vi "Run Contest.vi"() -> ()   [LabVIEW 2014]
uses:
  Participant.ctl
  Problem.ctl
  State Machine.ctl
  User Score Update.ctl
  Change Detect/Change Detect Int.vi
  Change Detect/Change Detect Boolean.vi
panel:
  in  "Update Ratings":bool
  in  "Early Finish":bool
  in  "Export Results":bool
  in  "Participant Names":string[](array[string])
  in  "Contest Length (hours)":dbl
  in  "Problem E Base Value":dbl=2500.0
  in  "Problem D Base Value":dbl=2000.0
  in  "Problem C Base Value":dbl=1500.0
  in  "Problem B Base Value":dbl=1000.0
  in  "Problem A Base Value":dbl=500.0
  in  "OK Button":bool
  in  "Problem":T1
  in  "Participant":string
  in  "At Time Remaining":dbl=3600.0
  out "Participant Status":T2[](array[typedef])
  in  "Participants":dbl
  in  "Contest Start":bool
  out "Time Remaining":u32
  out "Contest Indicator":bool
  out "Problem E Current Value":dbl
  out "Problem D Current Value":dbl
  out "Problem C Current Value":dbl
  out "Problem B Current Value":dbl
  out "Problem A Current Value":dbl
  # "You must export before starting a new Contest"
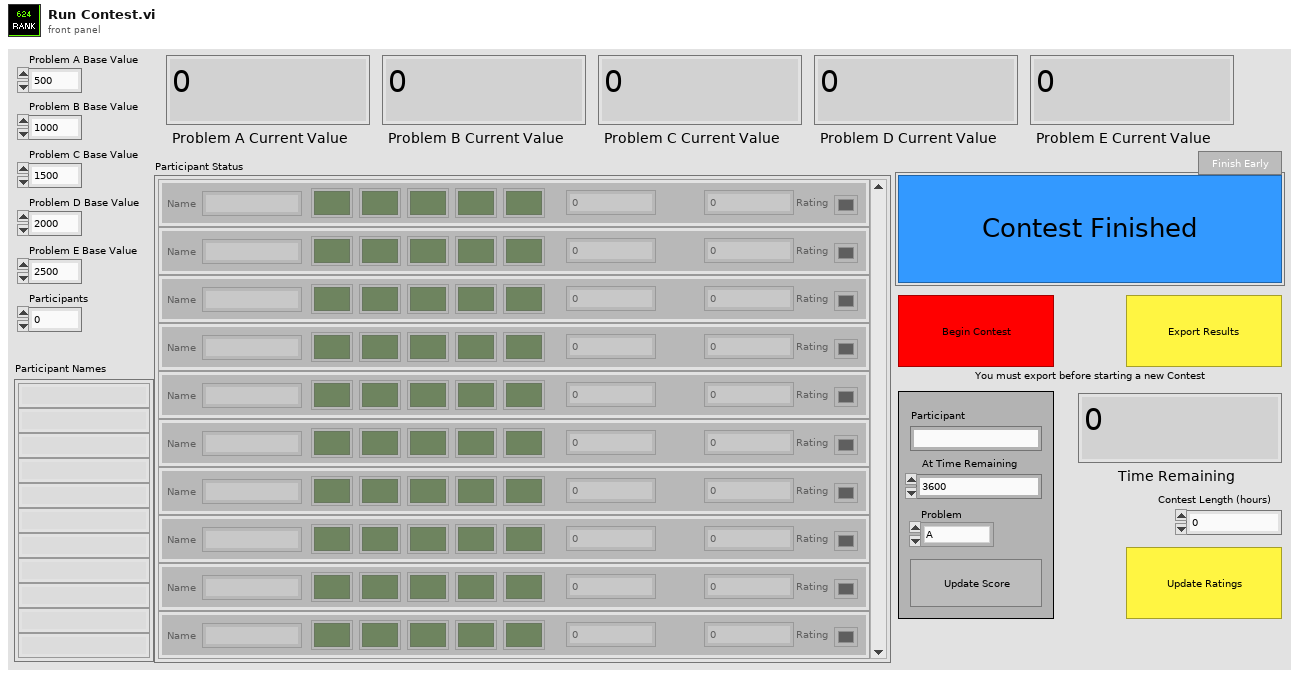
[diagram p1: front panel]
types:
  T1 = typedef "Problem.ctl" = enum16{"A", "B", "C", "D", "E"}
  T2 = typedef "Participant.ctl" = cluster{"Name":string, "A":bool, "Score":dbl, "B":bool, "C":bool, "D":bool, "E":bool, "Rating":dbl, "Color Box":u32}
  T3 = typedef "State Machine.ctl" = enum16{"Finish Contest", "Run Contest", "Begin Contest", "Wait for Start"}
  T4 = typedef "User Score Update.ctl" = cluster{"Score":dbl, "Name":string}
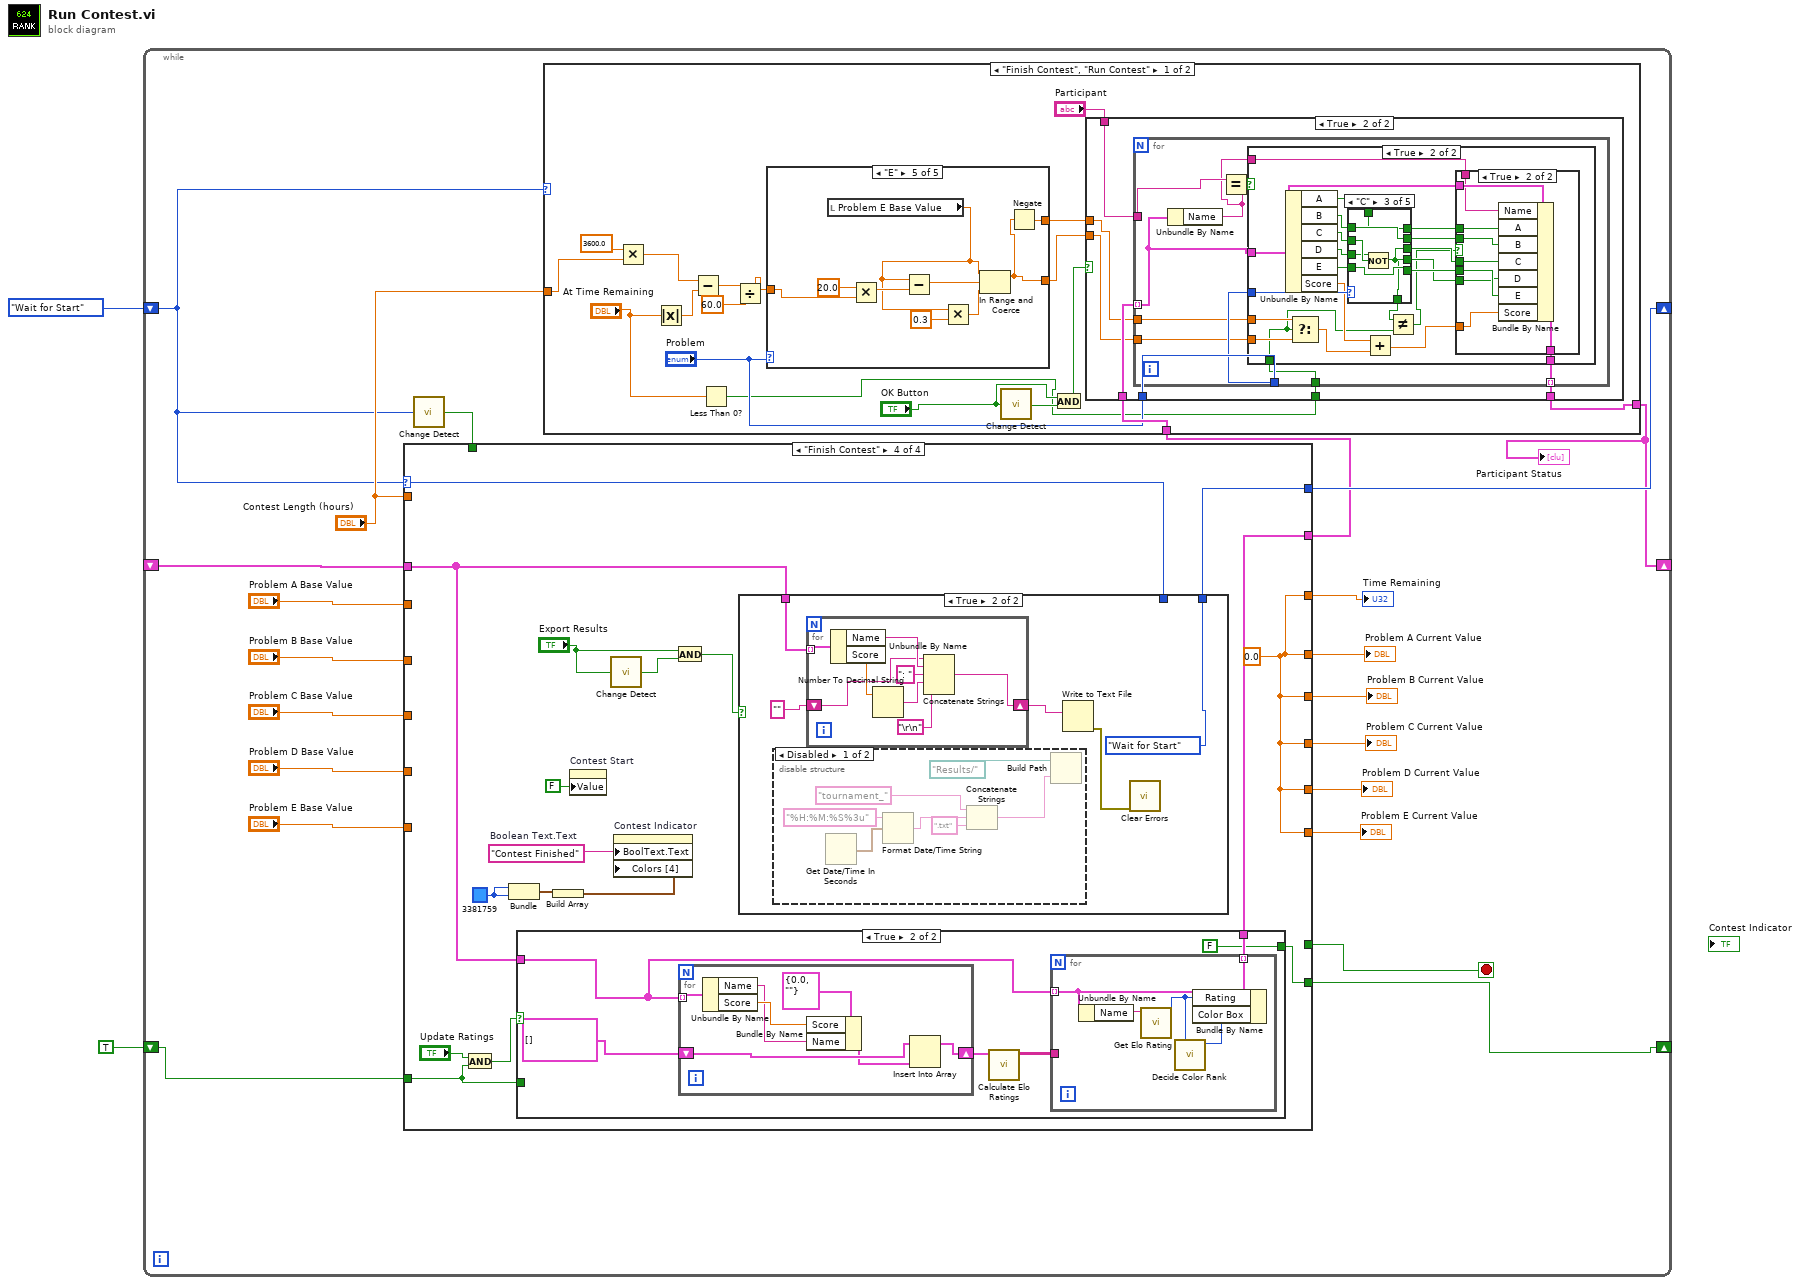
[diagram p0: block diagram]
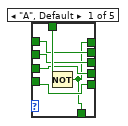
[diagram p5: hidden frame]
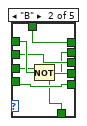
[diagram p6: hidden frame]
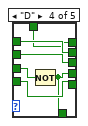
[diagram p7: hidden frame]
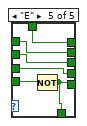
[diagram p8: hidden frame]
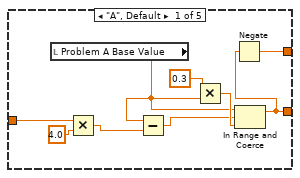
[diagram p9: hidden frame]
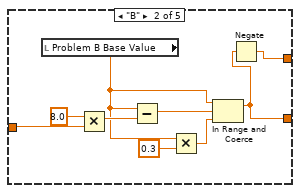
[diagram p10: hidden frame]
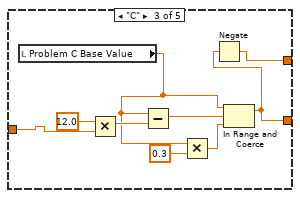
[diagram p11: hidden frame]
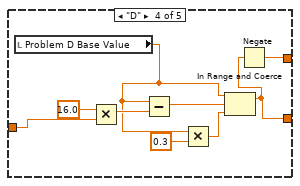
[diagram p12: hidden frame]
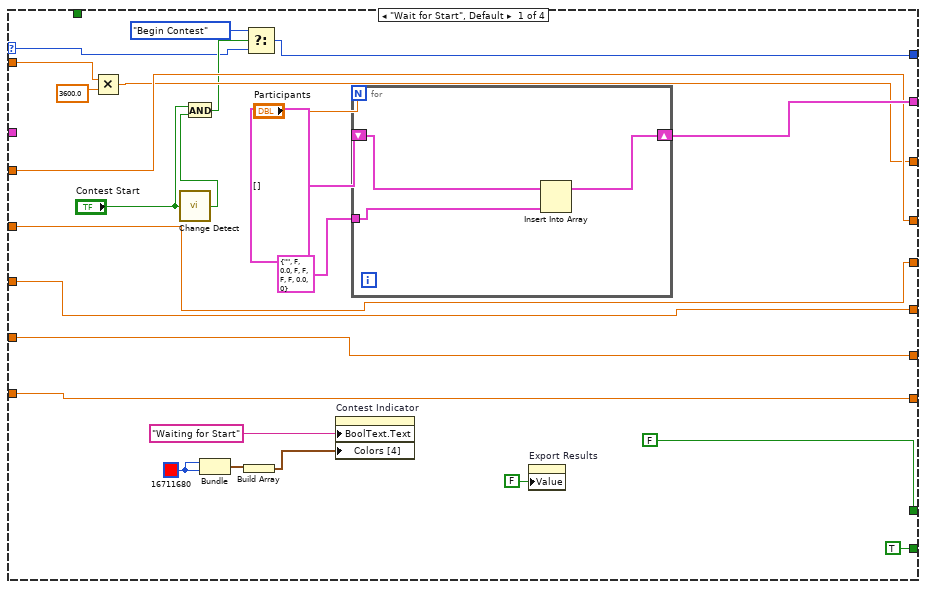
[diagram p14: hidden frame]
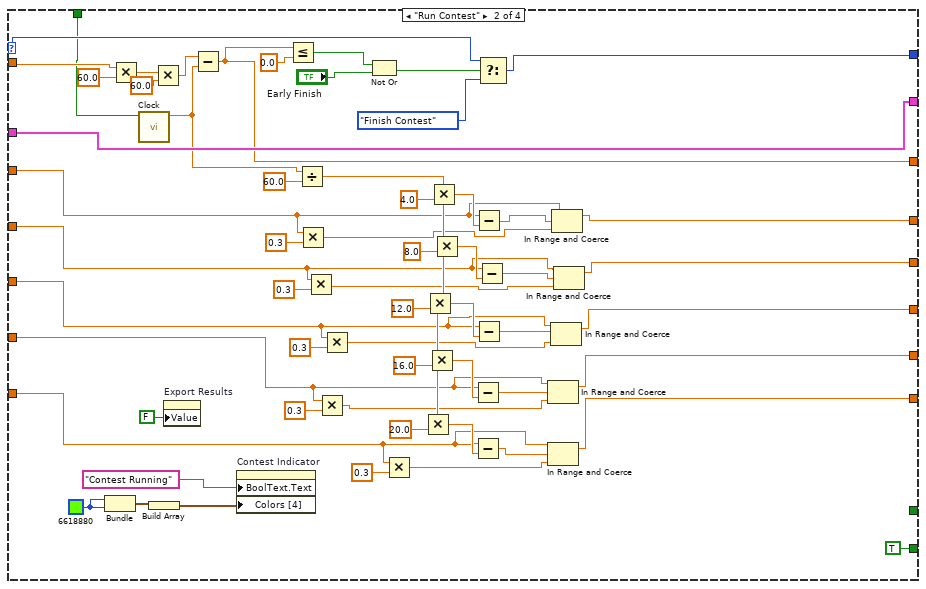
[diagram p15: hidden frame]
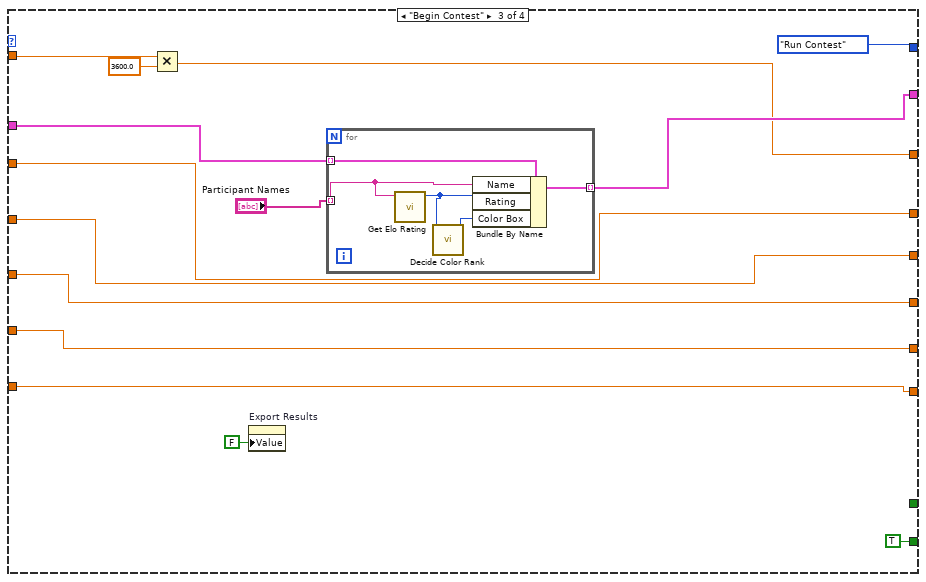
[diagram p16: hidden frame]
diagram:
  n1 = while {
    shift-right: [w6] -> _
    shift-left: _ -> [w22]
    shift-right: [w16] -> _
    shift-left: State_Machine."Wait for Start" -> [w5]
    shift-right: [w3] -> _
    shift-left: TRUE -> [w4]
    stop <- w23 stop-if-true
    n2 = call-poly "Change Detect.vi"("In"=w5) -> ("Changed?"=w9:bool)
    n3 = case shown="\"Finish Contest\"" w5 {
      selector: w5 -> [w170 w244 _ w282]
      tunnel: [FALSE _ _ _] -> w23
      tunnel: [w188 w242 w266 w278] -> w7
      tunnel: w22 -> [_ w242 w267 w279]
      tunnel: "Problem A Base Value" -> [w179 w227 w264 _]
      tunnel: "Problem B Base Value" -> [w180 w219 w263 _]
      tunnel: "Problem C Base Value" -> [w181 w216 w262 _]
      tunnel: "Problem D Base Value" -> [w182 w211 w261 _]
      tunnel: "Problem E Base Value" -> [w183 w208 w260 _]
      tunnel: "Contest Length (hours)" -> [w178 w246 w259 _]
      tunnel: [w169 w243 State_Machine."Run Contest" w281] -> w16
      tunnel: [w179 w228 w264 w286] -> w15
      tunnel: [w180 w217 w263 w286] -> w14
      tunnel: [w181 w213 w262 w286] -> w13
      tunnel: [w182 w209 w261 w286] -> w12
      tunnel: [w183 w205 w260 w286] -> w11
      tunnel: [w176 w204 w257 w286] -> w10
      tunnel: w9 -> [_ w203 _ _]
      tunnel: w4 -> [_ _ _ w274]
      tunnel: [TRUE TRUE TRUE w275] -> w3
      frame "Wait for Start", Default {
        w186 = u32 16711680
        n4 = Multiply(x=w178, y=3600.0) -> (x*y=w176:dbl)
        n5 = call-poly "Change Detect.vi"("In"="Contest Start") -> ("Changed?"=w173:bool)
        n6 = And(x="Contest Start", y=w173) -> (x .and. y?=w172:bool)
        n7 = Bundle(w186, w186) -> (w185:cluster{u32, u32})  [unwired: 1 in]
        n8 = Build Array(w185) -> (w184:cluster{u32, u32}[])
        n9 = Select(t=State_Machine."Begin Contest", s=w172, f=w170) -> (s? t:f=w169:T3)
        n10 = property on="Contest Indicator" class="Bool (strict)"("BoolText.Text"="Waiting for Start" ("Boolean Text.Text"), "Colors [4]"=w184) -> ()  [unwired: 2 in, 2 out]
        n11 = for {
          N: "Participants" -> [_]
          shift-right: [w195] -> w188
          shift-left: T2[] [] ("array") -> [w194]
          tunnel: T2 {"Name"="", "A"=FALSE, "Score"=0.0, "B"=FALSE, "C"=FALSE, "D"=FALSE, "E"=FALSE, "Rating"=0.0, "Color Box"=0} ("Participant") -> [w193]
          n12 = Insert Into Array(array=w194, new element=w193) -> (w195:T2[])  [unwired: 1 in]
        }
        n13 = property on="Export Results" class="Bool (strict)"("Value"=FALSE ("Export Results")) -> ()  [unwired: 2 in, 2 out]
      }
      frame "Run Contest" {
        w253 = u32 6618880
        n14 = Bundle(w253, w253) -> (w252:cluster{u32, u32})  [unwired: 1 in]
        n15 = Multiply(x=w246, y=60.0) -> (x*y=w248:dbl)
        n16 = call "Clock.vi"("Reset?"=w203) -> ("Time Elapsed"=w202:dbl)  [unwired: 10 in]
        n17 = Build Array(w252) -> (w251:cluster{u32, u32}[])
        n18 = Multiply(x=w248, y=60.0) -> (x*y=w250:dbl)
        n19 = property on="Export Results" class="Bool (strict)"("Value"=FALSE ("Export Results")) -> ()  [unwired: 2 in, 2 out]
        n20 = Subtract(x=w250, y=w202) -> (x-y=w204:dbl)
        n21 = property on="Contest Indicator" class="Bool (strict)"("BoolText.Text"="Contest Running" ("Boolean Text.Text"), "Colors [4]"=w251) -> ()  [unwired: 2 in, 2 out]
        n22 = Less Or Equal?(x=w204, y=0.0) -> (x <= y?=w200:bool)
        n23 = Divide(x=w202, y=60.0) -> (x/y=w240:dbl)
        n24 = Multiply(x=w227, y=0.3) -> (x*y=w225:dbl)
        n25 = Multiply(x=w219, y=0.3) -> (x*y=w218:dbl)
        n26 = Multiply(x=w211, y=0.3) -> (x*y=w210:dbl)
        n27 = Multiply(x=w216, y=0.3) -> (x*y=w215:dbl)
        n28 = Not Or(1:"Early Finish", 2:w200) -> (0:w199:bool)
        n29 = Multiply(x=w208, y=0.3) -> (x*y=w207:dbl)
        n30 = Multiply(x=w240, y=20.0) -> (x*y=w230:dbl)
        n31 = Multiply(x=w240, y=12.0) -> (x*y=w232:dbl)
        n32 = Multiply(x=w240, y=16.0) -> (x*y=w231:dbl)
        n33 = Multiply(x=w240, y=4.0) -> (x*y=w234:dbl)
        n34 = Multiply(x=w240, y=8.0) -> (x*y=w233:dbl)
        n35 = Subtract(x=w211, y=w231) -> (x-y=w212:dbl)
        n36 = Subtract(x=w208, y=w230) -> (x-y=w206:dbl)
        n37 = Subtract(x=w227, y=w234) -> (x-y=w229:dbl)
        n38 = Subtract(x=w216, y=w232) -> (x-y=w214:dbl)
        n39 = Subtract(x=w219, y=w233) -> (x-y=w220:dbl)
        n40 = Select(t=w244, s=w199, f=State_Machine."Finish Contest") -> (s? t:f=w243:T3)
        n41 = In Range and Coerce(upper limit=w211, x=w212, lower limit=w210) -> (coerced(x)=w209:dbl)  [unwired: 1 out]
        n42 = In Range and Coerce(upper limit=w208, x=w206, lower limit=w207) -> (coerced(x)=w205:dbl)  [unwired: 1 out]
        n43 = In Range and Coerce(upper limit=w216, x=w214, lower limit=w215) -> (coerced(x)=w213:dbl)  [unwired: 1 out]
        n44 = In Range and Coerce(upper limit=w227, x=w229, lower limit=w225) -> (coerced(x)=w228:dbl)  [unwired: 1 out]
        n45 = In Range and Coerce(upper limit=w219, x=w220, lower limit=w218) -> (coerced(x)=w217:dbl)  [unwired: 1 out]
      }
      frame "Begin Contest" {
        n46 = Multiply(x=w259, y=3600.0) -> (x*y=w257:dbl)
        n47 = property on="Export Results" class="Bool (strict)"("Value"=FALSE ("Export Results")) -> ()  [unwired: 2 in, 2 out]
        n48 = for {
          tunnel: w267 -> [w273] mode=indexing
          tunnel: "Participant Names" -> [w271] mode=indexing
          tunnel: [w272] -> w266 mode=indexing
          n49 = call "Get Elo Rating.vi"("Name"=w271) -> ("Rating"=w270:i32)  [unwired: 10 in]
          n50 = call "Decide Color Rank.vi"("Numeric"=w270) -> ("Color Box"=w269:u32)  [unwired: 10 in]
          n51 = Bundle By Name(cluster=w273, "Name"=w271, "Rating"=w270, "Color Box"=w269) -> (w272:T2)
        }
      }
      frame "Finish Contest" {
        w286 = 0.0 ("Problem A Base Value")
        w289 = u32 3381759
        w287 = "Contest Finished"  # Boolean Text.Text
        n52 = And(x="Update Ratings", y=w274) -> (x .and. y?=w276:bool)
        n53 = Bundle(w289, w289) -> (w290:cluster{u32, u32})  [unwired: 1 in]
        n54 = case shown="True" w276 {
          tunnel: w279 -> [w292 w295]
          tunnel: [w292 w294] -> w278
          tunnel: [w291 FALSE] -> w275
          tunnel: w274 -> [w291 _]
          frame False {
          }
          frame True {
            n55 = for {
              tunnel: w295 -> [w310] mode=indexing
              shift-right: [w304] -> w297
              shift-left: T4[] [] ("Names") -> [w306]
              n56 = Unbundle By Name(w310) -> ("Name"=w307:string, "Score"=w308:dbl)
              n57 = Bundle By Name(cluster=T4 {"Score"=0.0, "Name"=""} ("Score Update"), "Score"=w308, "Name"=w307) -> (w305:T4)
              n58 = Insert Into Array(array=w306, new element=w305) -> (w304:T4[])  [unwired: 1 in]
            }
            n59 = call "Calculate Elo Ratings.vi"("Names"=w297) -> ("Rating 2D Array"=w296:string[][])  [unwired: 8 in, 2 out]
            n60 = for {
              tunnel: w296 -> [_]
              tunnel: w295 -> [w303] mode=indexing
              tunnel: [w301] -> w294 mode=indexing
              n61 = Unbundle By Name(w303) -> ("Name"=w302:string)
              n62 = call "Get Elo Rating.vi"("Name"=w302) -> ("Rating"=w300:i32)  [unwired: 10 in]
              n63 = call "Decide Color Rank.vi"("Numeric"=w300) -> ("Color Box"=w299:u32)  [unwired: 10 in]
              n64 = Bundle By Name(cluster=w303, "Rating"=w300, "Color Box"=w299) -> (w301:T2)
            }
          }
        }
        n65 = Build Array(w290) -> (w288:cluster{u32, u32}[])
        n66 = property on="Contest Start" class="Bool (strict)"("Value"=FALSE ("Contest Start")) -> ()  [unwired: 2 in, 2 out]
        n67 = call-poly "Change Detect.vi"("In"="Export Results") -> ("Changed?"=w285:bool)
        n68 = property on="Contest Indicator" class="Bool (strict)"("BoolText.Text"=w287, "Colors [4]"=w288) -> ()  [unwired: 2 in, 2 out]
        n69 = And(x="Export Results", y=w285) -> (x .and. y?=w283:bool)
        n70 = case shown="True" w283 {
          tunnel: w279 -> [_ w316]
          tunnel: w282 -> [w311 _]
          tunnel: [w311 State_Machine."Wait for Start" ("f")] -> w281
          frame False {
          }
          frame True {
            n71 = disable-structure shown="Disabled" {
              frame Disabled {
                n72 = Get Date/Time In Seconds() -> (seconds since 1Jan1904=w322:timestamp)
                n73 = Format Date/Time String(time format string (%c)="%H:%M:%S%3u", seconds (now)=w322) -> (date/time string=w319:string)  [unwired: 1 in]
                n74 = Concatenate Strings("tournament_", w319, ".txt" ("string")) -> (w317:string)
                n75 = Build Path(base path=path "Results/", name or relative path=w317) -> ()  [unwired: 1 out]
              }
              frame Enabled {
              }
            }
            n76 = for {
              tunnel: w316 -> [w331] mode=indexing
              shift-right: [w324] -> w314
              shift-left: "" -> [w326]
              n77 = Unbundle By Name(w331) -> ("Name"=w330:string, "Score"=w328:dbl)
              n78 = Number To Decimal String(number=w328) -> (decimal integer string=w327:string)  [unwired: 1 in]
              n79 = Concatenate Strings(w326, w330, ": " ("string"), w327, "\r\n") -> (w324:string)
            }
            n80 = Write to Text File(text=w314) -> (error out=w313:errorcluster)  [unwired: 3 in, 2 out]
            n81 = call <vilib>:"Clear Errors.vi"("error in (no error)"=w313) -> ()  [unwired: 5 in, 2 out]
          }
        }
      }
    }
    "Problem A Current Value" <- w15
    "Problem B Current Value" <- w14
    "Problem C Current Value" <- w13
    "Problem D Current Value" <- w12
    "Problem E Current Value" <- w11
    "Time Remaining" <- w10
    n82 = case shown="\"Finish Contest\", \"Run Contest\"" w5 {
      tunnel: "Contest Length (hours)" -> [w40 _]
      tunnel: w7 -> [w33 w167]
      tunnel: [w31 w167] -> w6
      frame "Finish Contest", "Run Contest" {
        n83 = Multiply(x=3600.0, y=w40) -> (x*y=w39:dbl)
        n84 = Absolute Value(x="At Time Remaining") -> (abs(x)=w25:dbl)
        n85 = Subtract(x=w39, y=w25) -> (x-y=w30:dbl)
        n86 = Less Than 0?(x="At Time Remaining") -> (x < 0?=w27:bool)
        n87 = Divide(x=w30, y=60.0) -> (x/y=w29:dbl)
        n88 = case shown="\"E\"" "Problem" {
          tunnel: w29 -> [w129 w139 w143 w152 w161]
          tunnel: [w122 w131 w140 w149 w158] -> w35
          tunnel: [w123 w133 w142 w151 w160] -> w26
          frame "A", Default {
            n89 = local read "Problem A Base Value"() -> (w124:dbl)
            n90 = Multiply(x=w129, y=4.0) -> (x*y=w127:dbl)
            n91 = Subtract(x=w124, y=w127) -> (x-y=w125:dbl)
            n92 = Multiply(x=0.3 ("y"), y=w124) -> (x*y=w126:dbl)
            n93 = In Range and Coerce(upper limit=w124, x=w125, lower limit=w126) -> (coerced(x)=w122:dbl)  [unwired: 1 out]
            n94 = Negate(x=w122) -> (-x=w123:dbl)
          }
          frame "B" {
            n95 = local read "Problem B Base Value"() -> (w132:dbl)
            n96 = Multiply(x=8.0, y=w139) -> (x*y=w137:dbl)
            n97 = Subtract(x=w132, y=w137) -> (x-y=w136:dbl)
            n98 = Multiply(x=w132, y=0.3) -> (x*y=w134:dbl)
            n99 = In Range and Coerce(upper limit=w132, x=w136, lower limit=w134) -> (coerced(x)=w131:dbl)  [unwired: 1 out]
            n100 = Negate(x=w131) -> (-x=w133:dbl)
          }
          frame "C" {
            n101 = local read "Problem C Base Value"() -> (w141:dbl)
            n102 = Multiply(x=12.0, y=w143) -> (x*y=w147:dbl)
            n103 = Subtract(x=w141, y=w147) -> (x-y=w146:dbl)
            n104 = Multiply(x=w141, y=0.3) -> (x*y=w144:dbl)
            n105 = In Range and Coerce(upper limit=w141, x=w146, lower limit=w144) -> (coerced(x)=w140:dbl)  [unwired: 1 out]
            n106 = Negate(x=w140) -> (-x=w142:dbl)
          }
          frame "D" {
            n107 = local read "Problem D Base Value"() -> (w150:dbl)
            n108 = Multiply(x=16.0, y=w152) -> (x*y=w154:dbl)
            n109 = Subtract(x=w150, y=w154) -> (x-y=w155:dbl)
            n110 = Multiply(x=w150, y=0.3) -> (x*y=w157:dbl)
            n111 = In Range and Coerce(upper limit=w150, x=w155, lower limit=w157) -> (coerced(x)=w149:dbl)  [unwired: 1 out]
            n112 = Negate(x=w149) -> (-x=w151:dbl)
          }
          frame "E" {
            n113 = local read "Problem E Base Value"() -> (w159:dbl)
            n114 = Multiply(x=20.0, y=w161) -> (x*y=w163:dbl)
            n115 = Subtract(x=w159, y=w163) -> (x-y=w164:dbl)
            n116 = Multiply(x=w159, y=0.3) -> (x*y=w166:dbl)
            n117 = In Range and Coerce(upper limit=w159, x=w164, lower limit=w166) -> (coerced(x)=w158:dbl)  [unwired: 1 out]
            n118 = Negate(x=w158) -> (-x=w160:dbl)
          }
        }
        n119 = call-poly "Change Detect.vi"("In"="OK Button") -> ("Changed?"=w38:bool)
        n120 = And(x="OK Button", y=w38) -> (x .and. y?=w36:bool)
        n121 = case shown="True" w36 {
          tunnel: w35 -> [_ w46]
          tunnel: "Participant" -> [_ w48]
          tunnel: w33 -> [w42 w49]
          tunnel: "Problem" -> [_ w47]
          tunnel: [w42 w45] -> w31
          tunnel: w27 -> [_ w44]
          tunnel: w26 -> [_ w43]
          frame False {
          }
          frame True {
            n122 = for {
              tunnel: w49 -> [w55] mode=indexing
              tunnel: w48 -> [w57]
              tunnel: w47 -> [w58]
              tunnel: w46 -> [w54]
              tunnel: [w52] -> w45 mode=indexing
              tunnel: w44 -> [w51]
              tunnel: w43 -> [w50]
              n123 = Unbundle By Name(w55) -> ("Name"=w53:string)
              n124 = Equal?(x=w57, y=w53) -> (x = y?=w56:bool)
              n125 = case shown="True" w56 {
                tunnel: w58 -> [_ w81]
                tunnel: w55 -> [w59 w75]
                tunnel: w54 -> [_ w65]
                tunnel: w53 -> [_ w72]
                tunnel: [w59 w66] -> w52
                tunnel: w51 -> [_ w62]
                tunnel: w50 -> [_ w63]
                frame False {
                }
                frame True {
                  n126 = Unbundle By Name(w75) -> ("A"=w80:bool, "B"=w79:bool, "C"=w78:bool, "D"=w77:bool, "E"=w76:bool, "Score"=w74:dbl)
                  n127 = Select(t=w63, s=w62, f=w65) -> (s? t:f=w64:dbl)
                  n128 = case shown="\"C\"" w81 {
                    tunnel: w80 -> [w97 w102 w107 w111 w120]
                    tunnel: w79 -> [w96 w103 w108 w112 w119]
                    tunnel: w78 -> [w95 w101 w109 w113 w118]
                    tunnel: w77 -> [w94 w100 w106 w115 w117]
                    tunnel: w76 -> [w93 w99 w105 w114 w121]
                    tunnel: [w93 w99 w105 w114 w116] -> w71
                    tunnel: [w92 w102 w107 w111 w120] -> w67
                    tunnel: [w96 w98 w108 w112 w119] -> w68
                    tunnel: [w95 w101 w104 w113 w118] -> w69
                    tunnel: [w94 w100 w106 w110 w117] -> w70
                    tunnel: [w92 w98 w104 w110 w116] -> w61
                    frame "A", Default {
                      n129 = Not(x=w97) -> (.not. x?=w92:bool)
                    }
                    frame "B" {
                      n130 = Not(x=w103) -> (.not. x?=w98:bool)
                    }
                    frame "C" {
                      n131 = Not(x=w109) -> (.not. x?=w104:bool)
                    }
                    frame "D" {
                      n132 = Not(x=w115) -> (.not. x?=w110:bool)
                    }
                    frame "E" {
                      n133 = Not(x=w121) -> (.not. x?=w116:bool)
                    }
                  }
                  n134 = Add(x=w74, y=w64) -> (x+y=w73:dbl)
                  n135 = Not Equal?(x=w61, y=w62) -> (x != y?=w60:bool)
                  n136 = case shown="True" w60 {
                    tunnel: w75 -> [w82 w91]
                    tunnel: w73 -> [_ w89]
                    tunnel: w72 -> [_ w90]
                    tunnel: w71 -> [_ w88]
                    tunnel: w70 -> [_ w87]
                    tunnel: w69 -> [_ w86]
                    tunnel: w68 -> [_ w85]
                    tunnel: w67 -> [_ w84]
                    tunnel: [w82 w83] -> w66
                    frame False {
                    }
                    frame True {
                      n137 = Bundle By Name(cluster=w91, "Name"=w90, "A"=w84, "B"=w85, "C"=w86, "D"=w87, "E"=w88, "Score"=w89) -> (w83:T2)
                    }
                  }
                }
              }
            }
          }
        }
      }
      frame "Begin Contest", Default {
      }
    }
    "Participant Status" <- w6
  }
